vi "MyNoteTaker.vi"() -> ()   [LabVIEW 2013]
doc: "TC-1 Program to control Simple Step Boards v1.9"
panel:
  out "refnum out":refnum<file>
  out "Numeric":i32=122
  in  "Tab Control":enum32{"PDF VIEW", "Notes"}(tab)=enum."Notes"
  in  "Select PDF file":path
  in  "Open PDF":bool
  in  "PDF WINDOW":refnum<k7>(container)
  in  "Select text file":path
  in  "MY NOTES":string
  in  "SAVE":bool
  in  "CLOSE":bool
  in  "file operations":T1(ring)
  in  "Confirm":bool
  # "\"Ctrl + h\" : Enables helpful description information via context window"
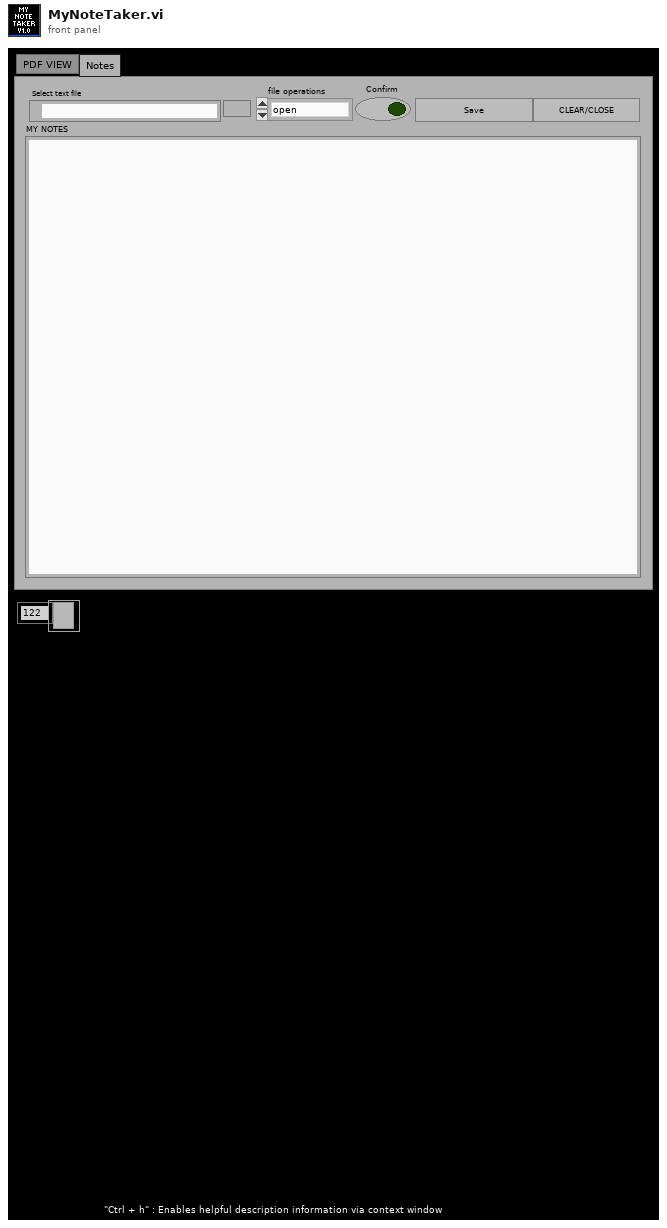
[diagram p1: front panel]
types:
  T1 = enum16{"open", "replace", "create", "open or create", "replace or create", "replace or create with confirmation"}
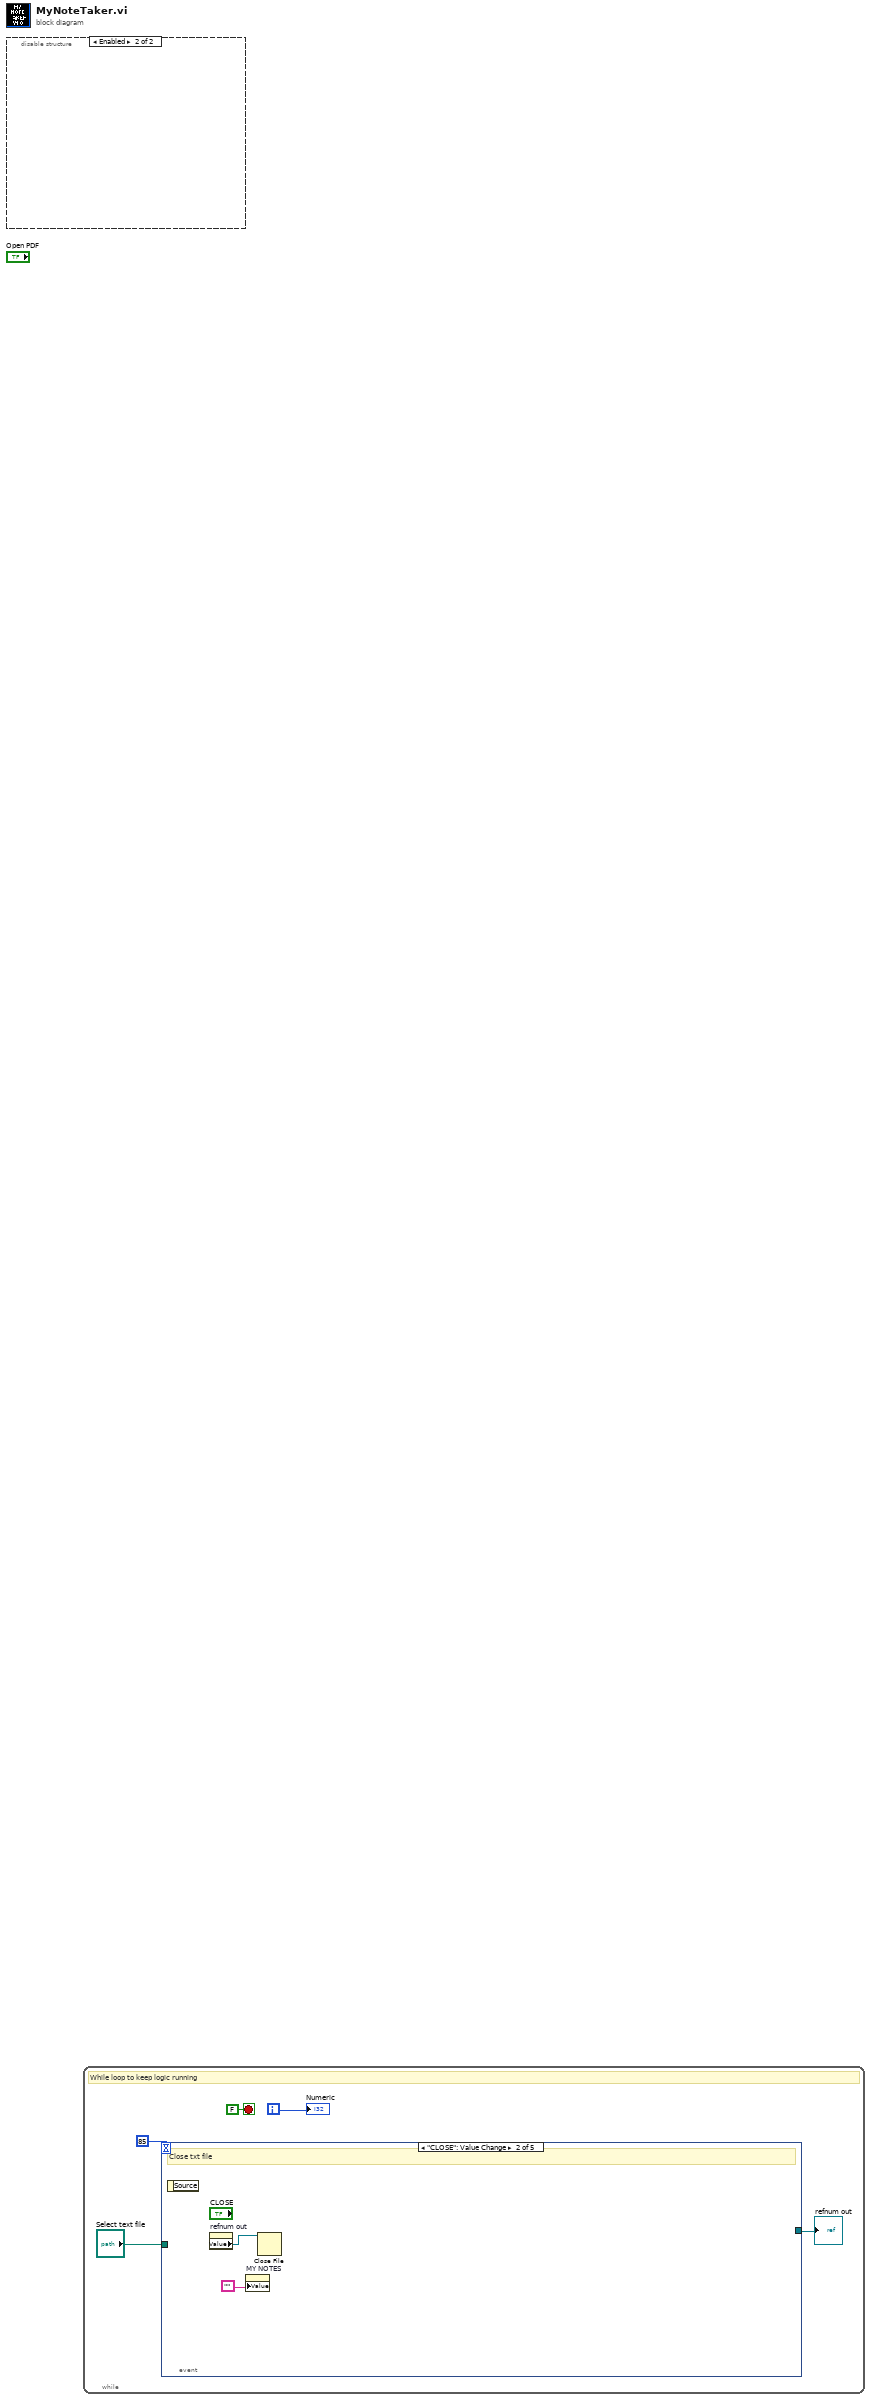
[diagram p0: block diagram]
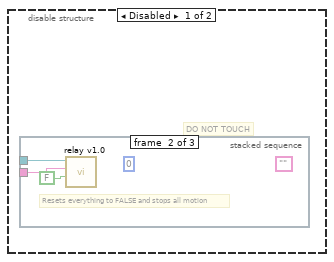
[diagram p2: hidden frame]
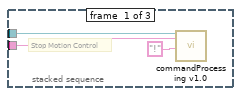
[diagram p3: hidden frame]
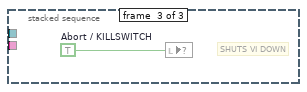
[diagram p4: hidden frame]
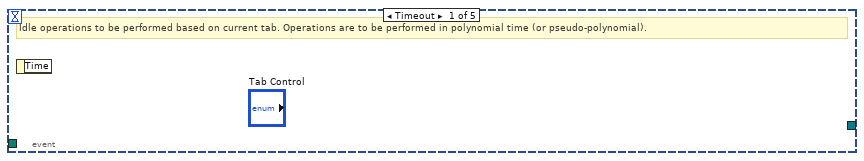
[diagram p5: hidden frame]
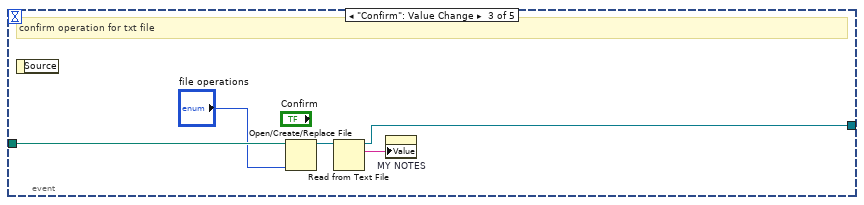
[diagram p6: hidden frame]
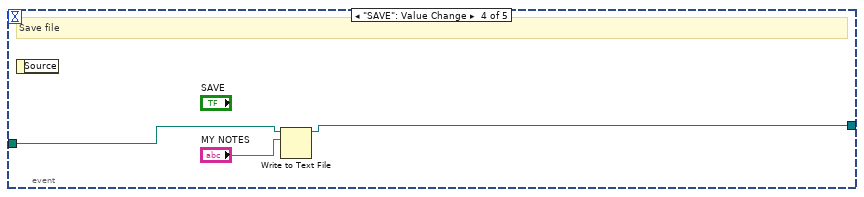
[diagram p7: hidden frame]
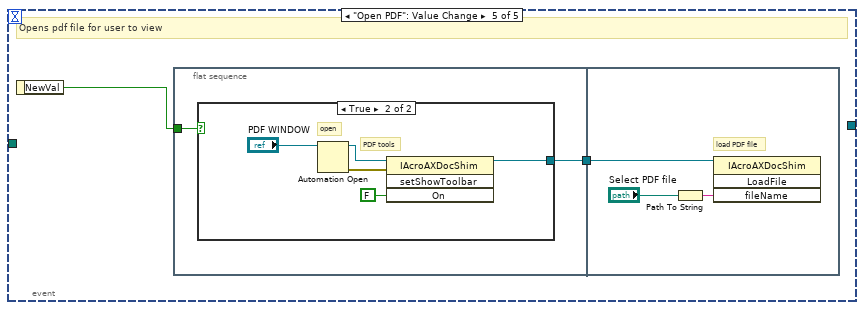
[diagram p8: hidden frame]
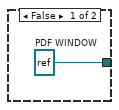
[diagram p9: hidden frame]
diagram:
  n1 = disable-structure shown="Enabled" {
    frame Disabled {
      # "DO NOT TOUCH"
      # "Resets everything to FALSE and stops all motion"
      n2 = stacked-sequence {
        tunnel: _ -> [w3 w6 _]
        tunnel: _ -> [w1 w5 _]
        frame #0 {
          # "Stop Motion Control"
          n3 = call "commandProcessing v1.0.vi"("Controller's Port"=w3, "Axis & Address"=w1, "Command"="!") -> ()  [unwired: 14 in, 3 out]
        }
        frame #1 {
          w7 = ""
          w8 = 0
          n4 = call "relay v1.0.vi"("Activate/Deactivate Relay"=FALSE, "Address"=w5, "Network Port"=w6) -> ()  [unwired: 9 in]
        }
        frame #2 {
          w9 = TRUE  # Abort / KILLSWITCH
          # "SHUTS VI DOWN"
          n5 = local write item#-1(w9) -> ()
        }
      }
    }
    frame Enabled {
    }
  }
  n6 = while {
    i -> [w11]
    stop <- FALSE stop-if-true
    # "While loop to keep logic running"
    n7 = event shown="[1] \"CLOSE\": Value Change" {
      selector: _ -> [_ _ _ _ _]
      dyn-events: _ -> [_ _ _ _ _]
      timeout: 85 -> [_ _ _ _ _]
      tunnel: "Select text file" -> [_ _ w19 w23 _]
      tunnel: [_ _ w17 w22 _] -> w10
      event Timeout {
        # "Idle operations to be performed based on current tab. Operations are to be performed in polynomial time (or pseudo-polynomial)."
        n8 = event-data() -> ()  [unwired: 1 in, 1 out]
      }
      event "CLOSE": Value Change {
        # "Close txt file"
        n9 = event-data() -> ()  [unwired: 1 in, 1 out]
        n10 = property on="refnum out" class="Ref (strict)"() -> ("Value"=w16:refnum<file>)  [unwired: 2 in, 2 out]
        n11 = property on="MY NOTES" class="Str"("Value"="") -> ()  [unwired: 2 in, 2 out]
        n12 = Close File(refnum=w16) -> ()  [unwired: 1 in, 2 out]
      }
      event "Confirm": Value Change {
        # "confirm operation for txt file"
        n13 = event-data() -> ()  [unwired: 1 in, 1 out]
        n14 = Open/Create/Replace File(file path (use dialog)=w19, operation (0:open)="file operations") -> (refnum out=w20:refnum<file>)  [unwired: 4 in, 2 out]
        n15 = Read from Text File(file (use dialog)=w20) -> (refnum out=w17:refnum<file>, text=w21:string)  [unwired: 3 in, 2 out]
        n16 = property on="MY NOTES" class="Str"("Value"=w21) -> ()  [unwired: 2 in, 2 out]
      }
      event "SAVE": Value Change {
        # "Save file"
        n17 = event-data() -> ()  [unwired: 1 in, 1 out]
        n18 = Write to Text File(file (use dialog)=w23, text="MY NOTES") -> (refnum out=w22:refnum<file>)  [unwired: 2 in, 2 out]
      }
      event "Open PDF": Value Change {
        # "Opens pdf file for user to view"
        n19 = event-data() -> ("NewVal"=w25:bool)  [unwired: 1 in]
        n20 = flat-sequence {
          tunnel: [w28] -> w26
          tunnel: w25 -> [w27]
          tunnel: w26 -> [w35]
          frame #0 {
            n21 = case shown="True" w27 {
              tunnel: [w29 w32] -> w28
              frame False {
                w29 = refnum<k7> refnum  # PDF WINDOW
              }
              frame True {
                # "open"
                # "PDF tools"
                n22 = Automation Open(Automation Refnum="PDF WINDOW") -> (Automation Refnum=w34:refnum<k7>, error out=w31:errorcluster)  [unwired: 3 in]
                n23 = invoke class="IAcroAXDocShim" method="setShowToolbar"(reference=w34, error in=w31, "On"=FALSE) -> (reference out=w32:refnum<k7>)  [unwired: 1 in, 3 out]
              }
            }
          }
          frame #1 {
            # "load PDF file"
            n24 = Path To String(path="Select PDF file") -> (string=w36:string)
            n25 = invoke class="IAcroAXDocShim" method="LoadFile"(reference=w35, "fileName"=w36) -> ()  [unwired: 2 in, 4 out]
          }
        }
      }
    }
    "refnum out" <- w10
    "Numeric" <- w11
  }
